vi "MListbox Replace Row.vi"(8 "error in (no error)":errorcluster, 9 "Row":string[](array[string]), 10 "Row Inex":u16, 11 "Multicolumn ListBox in":refnum<class "Multicolumn ListBox.lvclass">) -> (0 "error out":errorcluster, 3 "Multicolumn ListBox out":refnum<class "Multicolumn ListBox.lvclass">)   [LabVIEW 2012, in "Multicolumn ListBox.lvclass"]
uses:
  Multicolumn ListBox.lvclass
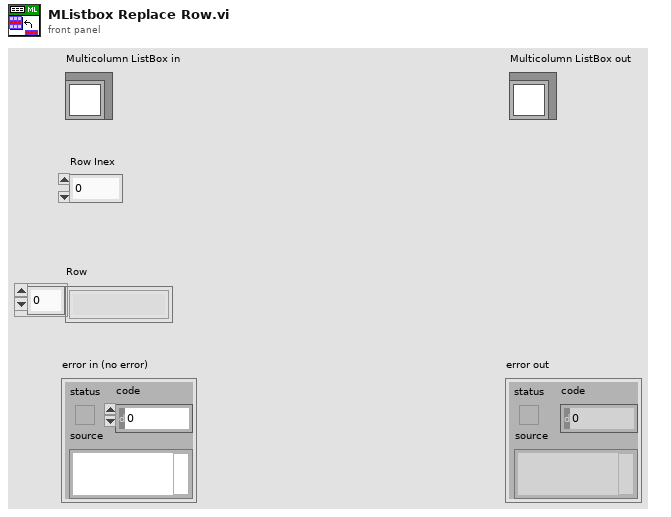
[diagram p1: front panel]
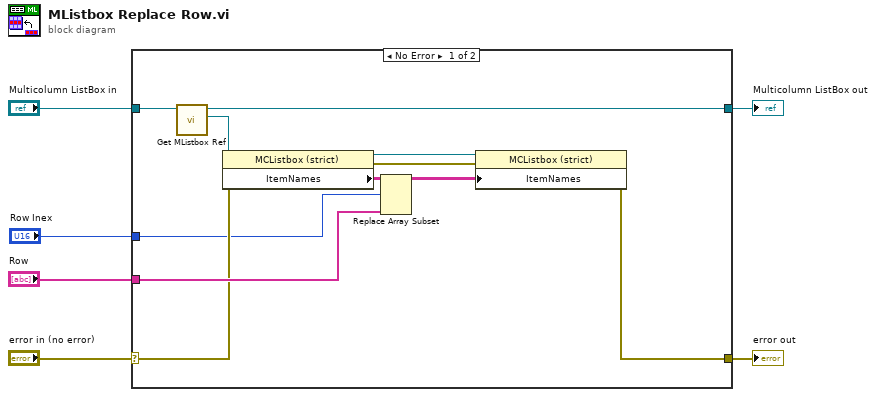
[diagram p0: block diagram]
diagram:
  n1 = case shown="No Error" "error in (no error)" {
    selector: "error in (no error)" -> [w9 w19]
    tunnel: [w8 w19] -> w5
    tunnel: [w16 w18] -> w3
    tunnel: "Multicolumn ListBox in" -> [w17 w18]
    tunnel: "Row Inex" -> [w7 _]
    tunnel: "Row" -> [w13 _]
    frame No Error {
      n2 = call "Get MListbox Ref.vi"("Multicolumn ListBox in"=w17) -> ("MListbox Ref"=w15:refnum<vi>, "Multicolumn ListBox out"=w16:refnum<class "Multicolumn ListBox.lvclass">)  [unwired: 8 in, 1 out]
      n3 = property class="MCListbox (strict)"(reference=w15, error in=w9) -> (reference out=w12:refnum<vi>, error out=w10:errorcluster, "ItemNames"=w14:string[][])
      n4 = Replace Array Subset(array=w14, new element=w13, index (row)=w7) -> (w11:string[][])  [unwired: 1 in]
      n5 = property class="MCListbox (strict)"(reference=w12, error in=w10, "ItemNames"=w11) -> (error out=w8:errorcluster)  [unwired: 1 out]
    }
    frame Error {
    }
  }
  "error out" <- w5
  "Multicolumn ListBox out" <- w3
